vi "Process.vi"(8 "error in (no error)":errorcluster, 10 "Pound in":refnum<class "Pound.lvclass">, 11 "Qbus in":refnum<class "Qbus.lvclass">) -> (0 "error out":errorcluster)   [LabVIEW 2017, in "McsaStartupAnalysis.lvlib"]
doc: "Measures additional startup-related features and writes the results to data events. If your users do not require startup features, you can omit this process from your device software."
uses:
  <vilib>/addons/InsightCM/Devices/Shared/Mcsa/McsaStartupAnalysis/McsaStartupAnalysis.lvlib
  <vilib>/addons/Qbus/Qbus.lvclass
  <vilib>/NI/Software Watchdog/Pound/Pound.lvclass
  <vilib>/addons/InsightCM/Devices/Shared/Mcsa/McsaStartupAnalysis/controls/Config.ctl
  <vilib>/addons/InsightCM/Devices/Shared/Mcsa/McsaStartupAnalysis/controls/Group.ctl
  <vilib>/addons/InsightCM/Devices/Shared/Mcsa/McsaStartupAnalysis/controls/ChannelForStartup.ctl
  <vilib>/addons/InsightCM/Devices/Shared/Mcsa/McsaStartupAnalysis/controls/StartupFeature.ctl
  <vilib>/addons/InsightCM/Devices/Shared/Mcsa/McsaStartupAnalysis/controls/MotorInfo.ctl
  <vilib>/NI/Software Watchdog/Watchdog/Watchdog.lvclass
  <vilib>/addons/InsightCM/Utilities/GlobalConfiguration/GlobalConfiguration.lvlib
  <vilib>/addons/InsightCM/Devices/Shared/Common/FileFlow/FileFlow.lvlib
  <vilib>/addons/TraceLogger/TraceLogger.lvlib
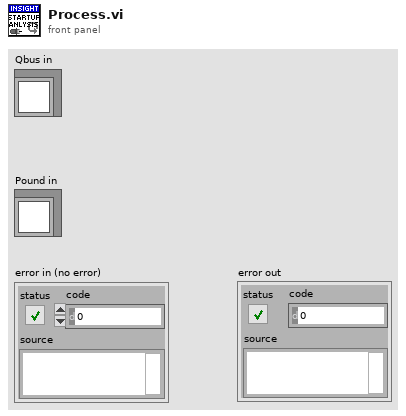
[diagram p1: front panel]
types:
  T1 = typedef "McsaStartupAnalysis.lvlib/Config.ctl" = cluster{"Groups":T2[]}
  T2 = typedef "McsaStartupAnalysis.lvlib/Group.ctl" = cluster{"Name":string, "Channels":T3[]}
  T3 = typedef "McsaStartupAnalysis.lvlib/ChannelForStartup.ctl" = cluster{"Name":string, "Id":string, "Type":string, "EnterStartupPFLA%":dbl, "ExitStartupPFLA%":dbl, "Features":T4[], "Motor Info":T5}
  T4 = typedef "McsaStartupAnalysis.lvlib/StartupFeature.ctl" = cluster{"MetricType":string, "Tag Id":string}
  T5 = typedef "McsaStartupAnalysis.lvlib/MotorInfo.ctl" = cluster{"Phase A AssetID":string, "Phase B AssetID":string, "Phase C AssetID":string, "Nominal Frequency":dbl, "Full Load Amps":dbl}
  T6 = typedef "FileFlow.lvlib/data_eventRef.ctl" = cluster{"event reference":T7, "DataGroup":string, "OperatingState":string, "StreamId":string, "LastBlock":bool, "Map":T8, "TrendPoints Only":bool, "Extra Large File":bool}
  T7 = typedef "DataEvent.lvlib/EventReference.ctl" = refnum<data-value>
  T8 = typedef "PointValueMap.lvlib/PointMap.ctl" = refnum<data-value>
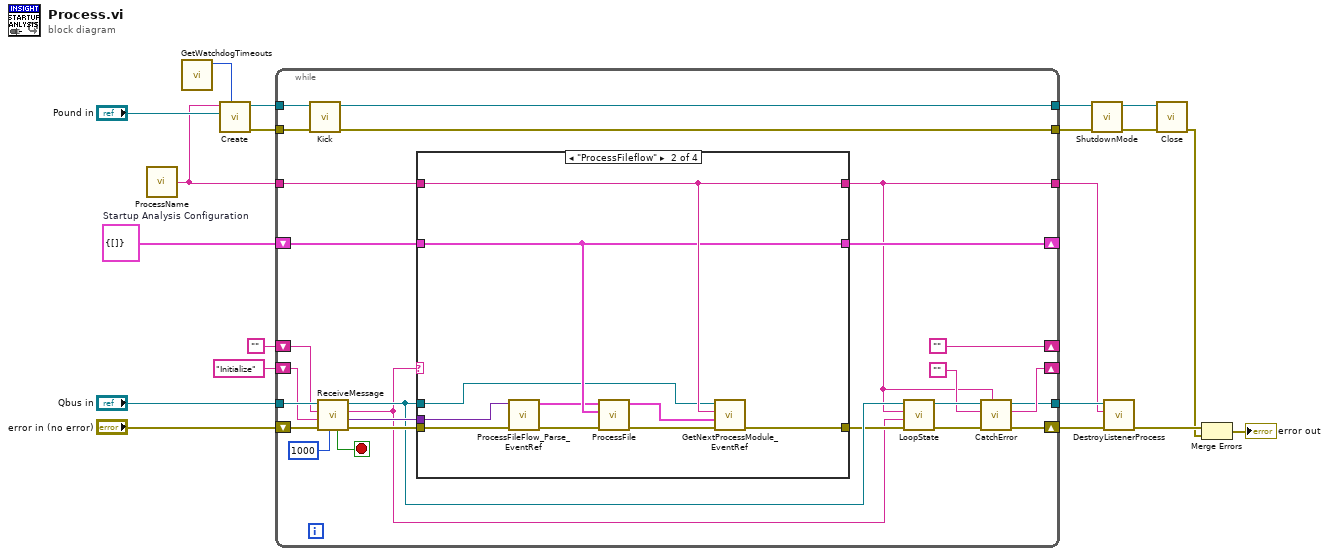
[diagram p0: block diagram]
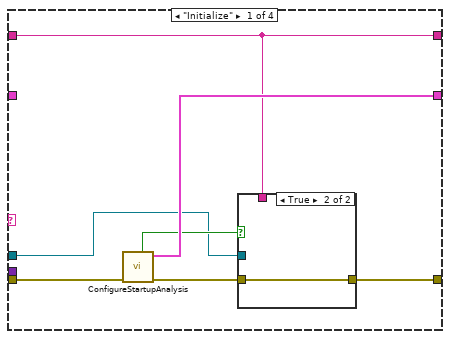
[diagram p2: hidden frame]
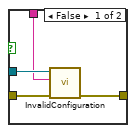
[diagram p3: hidden frame]
diagram:
  w2 = T1 {"Groups"=[]}  # Startup Analysis Configuration
  n1 = call <vilib>:"ProcessName.vi"() -> ("ProcessName"=w3:string)  [unwired: 5 in]
  n2 = call <vilib>:"GetWatchdogTimeouts.vi"() -> ("software timeout"=w1:u32)  [unwired: 10 in, 1 out]
  n3 = call <vilib>:"Create.vi"("Execution Timeout (ms)"=w1, "Pound"="Pound in", "Name"=w3) -> ("error out"=w10:errorcluster, "Watchdog"=w11:refnum<data-value>)  [unwired: 7 in]
  n4 = while {
    shift-right: [""] -> _
    shift-left: "" -> [w40]
    shift-right: [w46] -> _
    shift-left: w2 -> [w45]
    shift-right: [w27] -> _
    shift-left: "Initialize" ("MsgName") -> [w38]
    tunnel: w3 -> [w33]
    tunnel: [w26] -> w16
    tunnel: [w24] -> w15
    tunnel: "Qbus in" -> [w43]
    tunnel: [w37] -> w13
    tunnel: [w36] -> w12
    tunnel: w11 -> [w35]
    tunnel: w10 -> [w34]
    shift-right: [w25] -> w17
    shift-left: "error in (no error)" -> [w39]
    stop <- w22 stop-if-true
    n5 = call <vilib>:"Kick.vi"("error in (no error)"=w34, "Watchdog"=w35) -> ("error out"=w37:errorcluster, "Watchdog"=w36:refnum<data-value>)  [unwired: 8 in]
    n6 = call <vilib>:"ReceiveMessage.vi"("Timeout(100)"=1000, "error in (no error)"=w39, "Priority Action"=w38, "Default Action"=w40, "Qbus in"=w43) -> ("error out"=w41:errorcluster, "MsgValue"=w42:variant, "Action"=w23:string, "Qbus out"=w32:refnum<class "Qbus.lvclass">, "Exit"=w22:bool)  [unwired: 2 in]
    n7 = case shown="\"ProcessFileflow\"" w23 {
      tunnel: w41 -> [w53 w68 w70 w73]
      tunnel: [w50 w65 w70 w73] -> w31
      tunnel: w42 -> [_ w67 _ _]
      tunnel: [w52 w62 w69 w72] -> w46
      tunnel: w45 -> [_ w62 w69 w72]
      tunnel: w32 -> [w49 w60 _ _]
      tunnel: [w48 w66 w71 w74] -> w24
      tunnel: w33 -> [w48 w66 w71 w74]
      frame "Initialize" {
        n8 = call <vilib>:"ConfigureStartupAnalysis.vi"("error in (no error)"=w53) -> ("error out"=w47:errorcluster, "groups for startup measurement"=w52:T1, "valid config?"=w51:bool)  [unwired: 8 in]
        n9 = case shown="True" w51 {
          tunnel: [w56 w58] -> w50
          tunnel: w47 -> [w57 w58]
          tunnel: w49 -> [w55 _]
          tunnel: w48 -> [w54 _]
          frame False {
            n10 = call <vilib>:"InvalidConfiguration.vi"("error in (no error)"=w57, "description"=w54, "Qbus in"=w55) -> ("error out"=w56:errorcluster)  [unwired: 7 in, 1 out]
          }
          frame True {
          }
        }
      }
      frame "ProcessFileflow" {
        n11 = call <vilib>:"ProcessFileFlow_Parse_EventRef.vi"("error in (no error)"=w68, "body"=w67) -> ("error out"=w63:errorcluster, "data"=w59:T6)  [unwired: 8 in]
        n12 = call <vilib>:"ProcessFile.vi"("error in (no error)"=w63, "Startup Analysis Configuration"=w62, "data in"=w59) -> ("error out"=w61:errorcluster, "data out"=w64:T6)  [unwired: 7 in]
        n13 = call <vilib>:"GetNextProcessModule_EventRef.vi"("error in (no error)"=w61, "data"=w64, "source"=w66, "Qbus in"=w60) -> ("error out"=w65:errorcluster)  [unwired: 6 in, 1 out]
      }
      frame "Exit" {
      }
      frame "", Default {
      }
    }
    n14 = call <vilib>:"LoopState.vi"("error in (no error)"=w31, "loop action"=w23, "process name"=w24, "Qbus in"=w32) -> ("error out"=w28:errorcluster, "Qbus out"=w30:refnum<class "Qbus.lvclass">)  [unwired: 6 in]
    n15 = call <vilib>:"CatchError.vi"("source"=w24, "error in (no error)"=w28, "next action in"="", "Qbus in"=w30) -> ("error out"=w25:errorcluster, "next action out"=w27:string, "Qbus out"=w26:refnum<class "Qbus.lvclass">)  [unwired: 5 in]
  }
  n16 = call <vilib>:"ShutdownMode.vi"("error in (no error)"=w13, "Watchdog"=w12) -> ("error out"=w18:errorcluster, "Watchdog"=w19:refnum<data-value>)  [unwired: 8 in]
  n17 = call <vilib>:"DestroyListenerProcess.vi"("error in (no error)"=w17, "process name"=w15, "Qbus in"=w16) -> ("error in (no error)"=w9:errorcluster)  [unwired: 7 in, 1 out]
  n18 = call <vilib>:"Close.vi"("error in (no error)"=w18, "Watchdog"=w19) -> ("error out"=w8:errorcluster)  [unwired: 9 in]
  n19 = Merge Errors(w9, w8) -> (→"error out":errorcluster)
